vi "step.vi"(8 "error in (no error)":errorcluster, 11 "para0":u64) -> (0 "error out":errorcluster, 2 "sqlite3_step":i32, 3 "para0 out":u64)   [LabVIEW 2020, in "sqlite3.lvlib"]
uses:
  sqlite3.lvlib
  bin/sqlite3_64.dll
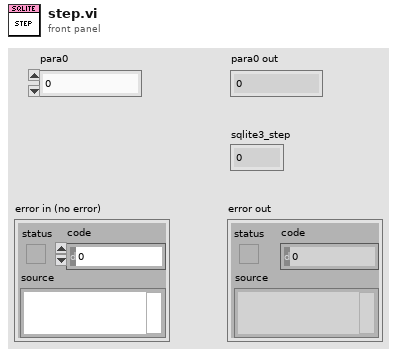
[diagram p1: front panel]
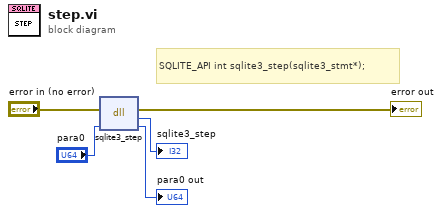
[diagram p0: block diagram]
diagram:
  # "SQLITE_API int sqlite3_step(sqlite3_stmt*);"
  n1 = dll-call lib="D:/Project/Labview-Projects/database-configuration/externals/sqlite3/Source/bin/sqlite3_*.*" fn="sqlite3_step"(error in="error in (no error)", "para0"="para0") -> (error out=→"error out":errorcluster, "return type"=→"sqlite3_step":i32, "para0"=→"para0 out":u64)  [unwired: 2 in, 1 out]
